vi "WheelShooter Shoot(Manual).vi"(4 "CollectSpeed(t/100ms)":dbl, 5 "Angle(degrees)":dbl, 6 "LaunchSpeed(t/100ms)":dbl, 7 "error in":errorcluster, 8 "Collection Trigger":bool, 9 "Spinup Trigger":bool, 10 "Trigger":bool) -> (0 "error out":errorcluster)   [LabVIEW 2015]
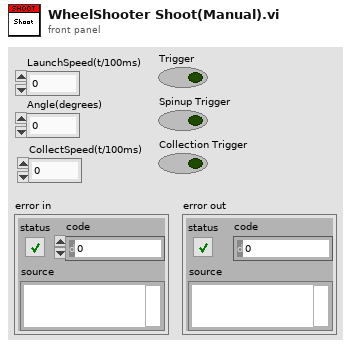
[diagram p1: front panel]
types:
  T1 = typedef "Firing Cluster.ctl" = cluster{"error":errorcluster, "AngleMotorRefnum":T2, "LeftWheelRefnum":T2, "RightWheelRefnum":T2, "PushSolenoidRefnum":T9, "AngleMotorPosition(t)":dbl, "LaunchSpeed(t/100ms)":dbl, "CollectSpeed(t/100ms)":dbl}
  T2 = typedef "WPI_MotorControlDeviceRef.ctl" = cluster{"DeviceStatus":errorcluster, "Type":T3, "PWM":cluster{"PWM Channel":T4, "DeadBand":T5}, "CAN":cluster{"Device Number":u8, "Control Mode":T6, "Semaphore":T7, "Max Vout":dbl, "TalonSRX Control Mode":T8}, "Invert":bool}
  T3 = typedef "WPI_MotorControlType.ctl" = enum16{"PWM", "CAN", "CANTalonSRX"}
  T4 = typedef "FPGA_DIOPWMChannel.ctl" = enum8{"PWM 0", "PWM 1", "PWM 2", "PWM 3", "PWM 4", "PWM 5", "PWM 6", "PWM 7", "PWM 8", "PWM 9", "PWM MXP 0", "PWM MXP 1", "PWM MXP 2", "PWM MXP 3", "PWM MXP 4", "PWM MXP 5", "PWM MXP 6", "PWM MXP 7", "PWM MXP 8", "PWM MXP 9", "Invalid"}
  T5 = typedef "WPI_PWMDeadband.ctl" = cluster{"Name":string, "maxPositivePwm":i32, "minPositivePwm":i32, "centerPwm":i32, "maxNegativePwm":i32, "minNegativePwm":i32, "angularRange":u16}
  T6 = typedef "WPI_CANJaguar_ControlMode.ctl" = enum8{"Percent VBus", "Current", "Speed", "Position", "Voltage"}
  T7 = typedef "Semaphore RefNum" = refnum<k1>
  T8 = typedef "WPI_CANTalonSRX_APIControlMode.ctl" = enum8{"Percent VBus", "Speed", "Position", "Slave", "Unchanged / Invalid", "Voltage Compensation", "Current", "Motion Profile"}
  T9 = typedef "WPI_SolenoidDevRef.ctl" = cluster{"DevStatus":errorcluster, "Pneumatics Control Module":u8, "Forward Solenoid Channel":T10, "Reverse Solenoid Channel":T10}
  T10 = typedef "WPI_SolenoidChannel.ctl" = enum8{"Solenoid 0", "Solenoid 1", "Solenoid 2", "Solenoid 3", "Solenoid 4", "Solenoid 5", "Solenoid 6", "Solenoid 7", "Invalid"}
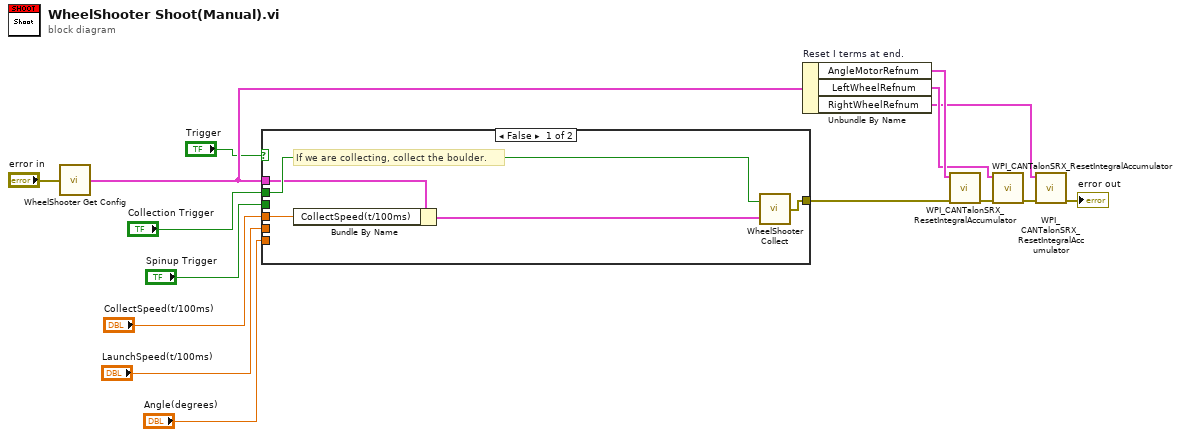
[diagram p0: block diagram]
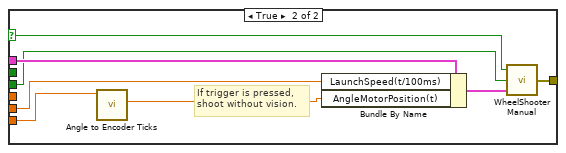
[diagram p2: hidden frame]
diagram:
  n1 = call "WheelShooter Get Config.vi"("error in"="error in") -> (0:w12:T1)
  n2 = case shown="False" "Trigger" {
    selector: "Trigger" -> [_ w25]
    tunnel: w12 -> [w17 w28]
    tunnel: [w19 w27] -> w8
    tunnel: "Collection Trigger" -> [w20 _]
    tunnel: "Spinup Trigger" -> [_ w24]
    tunnel: "LaunchSpeed(t/100ms)" -> [_ w23]
    tunnel: "Angle(degrees)" -> [_ w22]
    tunnel: "CollectSpeed(t/100ms)" -> [w18 _]
    frame False {
      # "If we are collecting, collect the boulder."
      n3 = Bundle By Name(cluster=w17, "CollectSpeed(t/100ms)"=w18) -> (w16:T1)
      n4 = call "WheelShooter Collect.vi"("Firing Data"=w16, "CollectionTrigger"=w20) -> ("error out"=w19:errorcluster)
    }
    frame True {
      # "If trigger is pressed,\nshoot without vision."
      n5 = call "Angle to Encoder Ticks.vi"("Angle(degrees)"=w22) -> ("Rotations"=w26:dbl)  [unwired: 10 in]
      n6 = Bundle By Name(cluster=w28, "LaunchSpeed(t/100ms)"=w23, "AngleMotorPosition(t)"=w26) -> (w21:T1)
      n7 = call "WheelShooter Manual.vi"("Firing Data"=w21, "Spinup Trigger"=w24, "Trigger"=w25) -> ("error out"=w27:errorcluster)
    }
  }
  n8 = Unbundle By Name "Reset I terms at end."(w12) -> ("AngleMotorRefnum"=w11:T2, "LeftWheelRefnum"=w10:T2, "RightWheelRefnum"=w9:T2)
  n9 = call <vilib>:"WPI_CANTalonSRX_ResetIntegralAccumulator.vi"("error in (no error)"=w8, "CAN Talon SRX Ref"=w11) -> ("error out"=w14:errorcluster)  [unwired: 8 in, 1 out]
  n10 = call <vilib>:"WPI_CANTalonSRX_ResetIntegralAccumulator.vi"("error in (no error)"=w14, "CAN Talon SRX Ref"=w10) -> ("error out"=w15:errorcluster)  [unwired: 8 in, 1 out]
  n11 = call <vilib>:"WPI_CANTalonSRX_ResetIntegralAccumulator.vi"("error in (no error)"=w15, "CAN Talon SRX Ref"=w9) -> ("error out"=→"error out":errorcluster)  [unwired: 8 in, 1 out]
